vi "Triggering External start.vi"(8 "error in (no error)":errorcluster, 10 "source":T1 items=["AO_Start", "AI_Start", "DSP_Start"], 11 "MicroDAQ.lvlib:Analog output.lvclass":refnum<class "Analog output.lvclass">) -> (0 "error out":errorcluster, 3 "MicroDAQ.lvlib:Analog output.lvclass out":refnum<class "Analog output.lvclass">)   [LabVIEW 2009, in "MicroDAQ.lvlib" / "Analog output.lvclass"]
doc: "With this trigger task will start when given other task starts processing."
uses:
  <instrlib>/MicroDAQ/Channel/Analog Output/Analog output.lvclass
  <instrlib>/MicroDAQ/Tools/External start trigger source.ctl
  <instrlib>/MicroDAQ/Tools/Trigger type.ctl
  <instrlib>/MicroDAQ/MicroDAQ.lvlib
  <instrlib>/MicroDAQ/Channel/Channel.lvclass
  <instrlib>/MicroDAQ/Mlink library wraper/mlink.lvlib
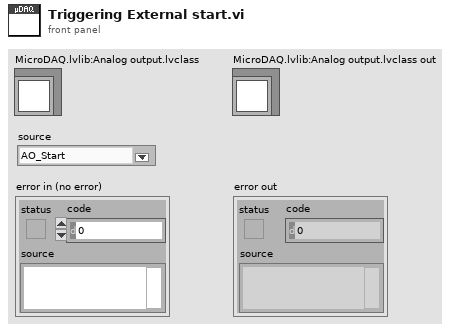
[diagram p1: front panel]
types:
  T1 = typedef "MicroDAQ.lvlib/External start trigger source.ctl" = u8
  T2 = typedef "MicroDAQ.lvlib/Trigger type.ctl" = enum8{"Analog output", "Analog input"}
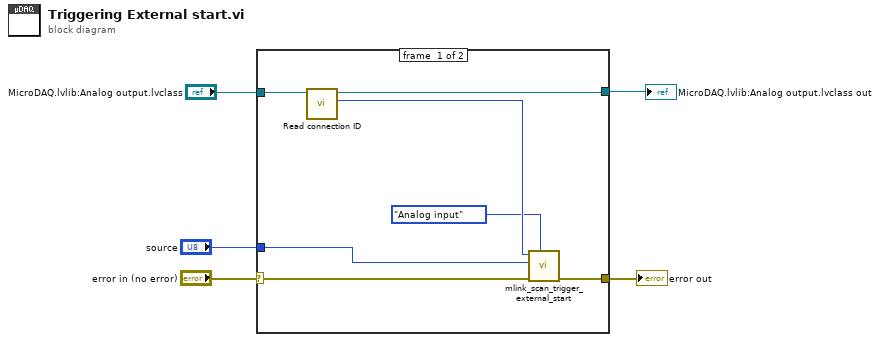
[diagram p0: block diagram]
diagram:
  n1 = case shown="No Error" "error in (no error)" {
    selector: "error in (no error)" -> [w10 w13]
    tunnel: [w9 w13] -> w4
    tunnel: [w11 w14] -> w2
    tunnel: "MicroDAQ.lvlib:Analog output.lvclass" -> [w12 w14]
    tunnel: "source" -> [w6 _]
    frame #0 {
      n2 = call <instrlib>:"Read connection ID.vi"("Task in"=w12) -> ("connection ID"=w8:i32, "Task out"=w11:refnum<class "Analog output.lvclass">)  [unwired: 9 in]
      n3 = call <instrlib>:"mlink_scan_trigger_external_start.vi"("trigger type"=Trigger_type."Analog input", "error in (no error)"=w10, "source"=w6, "connection ID"=w8) -> ("error out"=w9:errorcluster)  [unwired: 6 in, 1 out]
    }
    frame #1 {
    }
  }
  "error out" <- w4
  "MicroDAQ.lvlib:Analog output.lvclass out" <- w2
